vi "start Julia ZMQ server.vi"(8 "error in (no error)":errorcluster, 11 "Julia user functions script":path=path "C:/_LabView_projects/ZMQ/LV_ZMQ_Jl.jl/src/Julia/dummy.jl") -> (0 "error out":errorcluster, 1 "tmp file out":path, 2 "jl-script file out":path, 3 "return code":i32)   [LabVIEW 2018, in "LV-0mq-Julia_roundtrip-lib.lvlib" / "LV2Julia_core.lvlib"]
uses:
  LV2Julia_core.lvlib
  jl-scripts path.vi
panel:
  out "Julia script":string
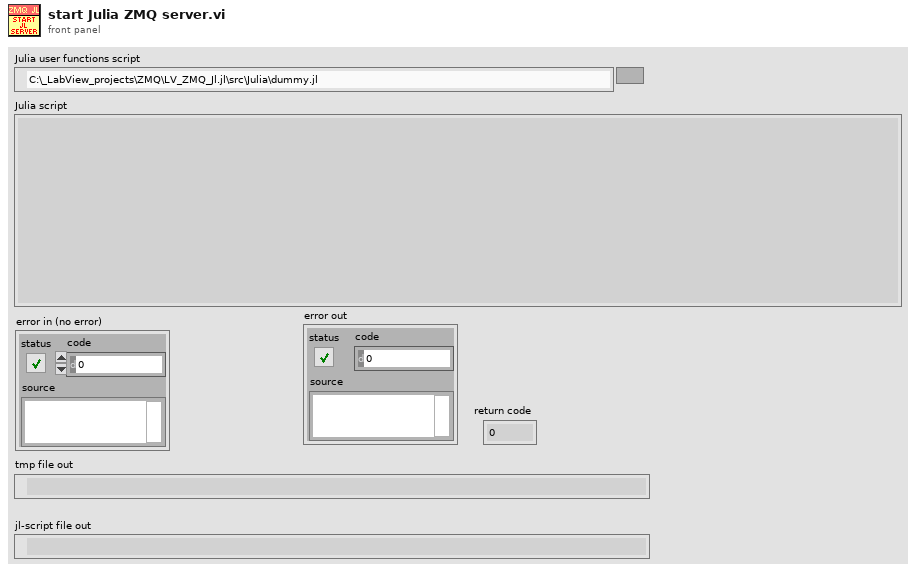
[diagram p1: front panel]
types:
  T1 = enum16{"open", "replace", "create", "open or create", "replace or create", "replace or create with confirmation"}
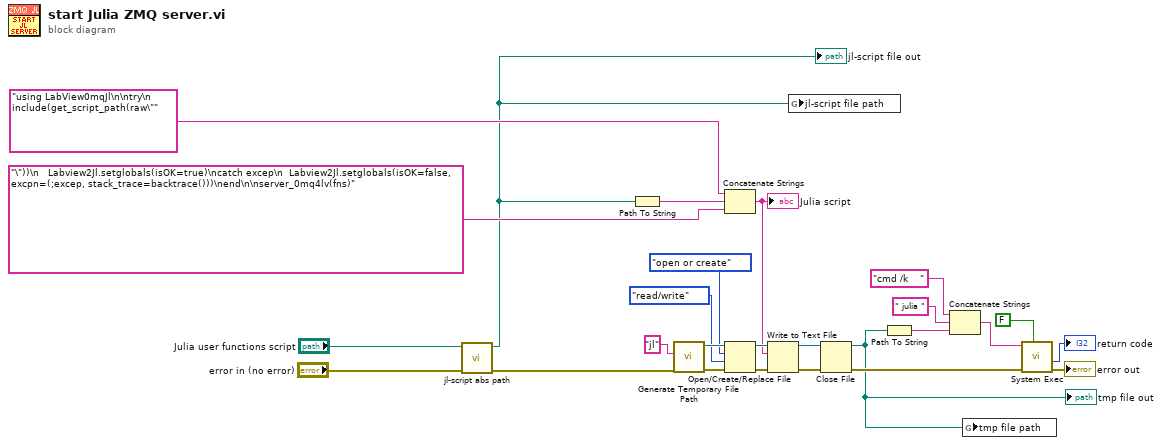
[diagram p0: block diagram]
diagram:
  n1 = call "jl-script abs path.vi"("error in (no error)"="error in (no error)", "Julia user functions script"="Julia user functions script") -> ("error out"=w5:errorcluster, "script abs path"=w2:path)  [unwired: 8 in]
  "jl-script file out" <- w2
  n2 = Path To String(path=w2) -> (string=w1:string)
  n3 = call <vilib>:"Generate Temporary File Path.vi"("error in (no error)"=w5, "Temporary File Extension (tmp)"="jl") -> ("error out"=w22:errorcluster, "Unique Temporary File Path"=w23:path)  [unwired: 8 in]
  n4 = Concatenate Strings("using LabView0mqJl\n\ntry\n   include(get_script_path(raw\"", w1, "\"))\n   Labview2Jl.setglobals(isOK=true)\ncatch excep\n  Labview2Jl.setglobals(isOK=false, excpn=(;excep, stack_trace=backtrace()))\nend\n\nserver_0mq4lv(fns)") -> (w17:string)
  "Julia script" <- w17
  n5 = Open/Create/Replace File(file path (use dialog)=w23, error in=w22, operation (0:open)=T1."open or create", access (0:read/write)=enum16{"read/write", "read-only", "write-only"}."read/write") -> (refnum out=w18:refnum<file>, error out=w19:errorcluster)  [unwired: 2 in, 1 out]
  n6 = Write to Text File(file (use dialog)=w18, text=w17, error in=w19) -> (refnum out=w16:refnum<file>, error out=w15:errorcluster)  [unwired: 1 in, 1 out]
  n7 = global write "jl-scripts path.vi" "jl-script file path"(w2) -> ()
  n8 = Close File(refnum=w16, error in=w15) -> (path=w4:path, error out=w7:errorcluster)
  "tmp file out" <- w4
  n9 = Path To String(path=w4) -> (string=w11:string)
  n10 = Concatenate Strings("cmd /k    ", " julia ", w11) -> (w10:string)
  n11 = global write "jl-scripts path.vi" "tmp file path"(w4) -> ()
  n12 = call <vilib>:"System Exec.vi"("wait until completion? (T)"=FALSE, "error in (no error)"=w7, "command line"=w10) -> ("error out"=→"error out":errorcluster, "return code"=→"return code":i32)  [unwired: 5 in, 2 out]
